vi "Handle Last Ack Core.vi"(4 "error in (no error)":errorcluster, 6 "Last Ack":refnum<class "Last Ack.lvclass">, 7 "Assert Startup UI in":refnum<class "Assert Startup UI.lvclass">) -> (0 "error out":errorcluster, 3 "Assert Startup UI out":refnum<class "Assert Startup UI.lvclass">)   [LabVIEW 2016, in "Assert Startup UI.lvlib" / "Assert Startup UI.lvclass"]
doc: "(<B>Filename</B>: Actor Framework.lvlib:Actor.lvclass:Handle Last Ack Core.vi)\n\nDefines how the caller actor responds to the Last Ack message from a nested actor. The Last Ack message is the final message a nested actor sends to its caller before it shuts down. The message contains information about the final state of the nested actor.\n\nBy default, this method does nothing except return any error the nested actor sent. A descendant class may override this method to define behavior."
uses:
  Assert Startup UI.lvclass
  <vilib>/ActorFramework/LastAck/Last Ack.lvclass
  Assert Startup UI.lvclass/Assert Startup UI.ctl
  Base UI Actor/Base UI Actor/Base UI Actor.lvclass
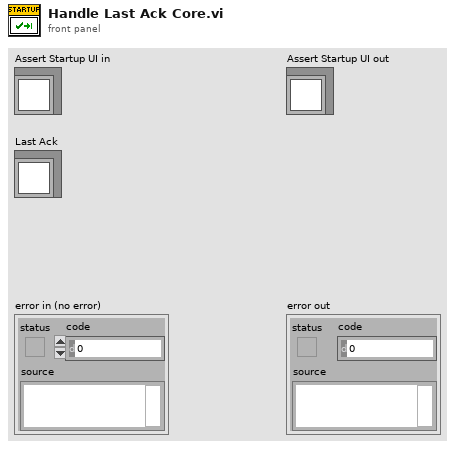
[diagram p1: front panel]
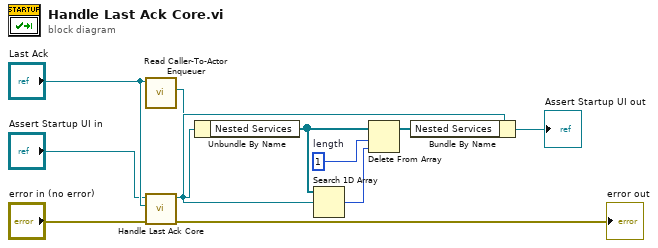
[diagram p0: block diagram]
diagram:
  w4 = 1  # length
  n1 = call <vilib>:"Read Caller-To-Actor Enqueuer.vi"("Last Ack"="Last Ack") -> ("Caller-to-Actor Enqueuer"=w6:refnum<class "Message Enqueuer.lvclass">)  [unwired: 10 in]
  n2 = call-parent "Handle Last Ack Core.vi"("error in (no error)"="error in (no error)", "Last Ack"="Last Ack", "Actor in"="Assert Startup UI in") -> ("error out"=→"error out":errorcluster, "Actor out"=w7:refnum<class "Assert Startup UI.lvclass">)  [unwired: 3 in]
  n3 = Unbundle By Name(w7) -> ("Nested Services"=w5:refnum<class "Message Enqueuer.lvclass">[])
  n4 = Search 1D Array(1D array=w5, element=w6) -> (index of element=w3:i32)  [unwired: 1 in]
  n5 = Delete From Array(array=w5, length=w4, index=w3) -> (array with subset deleted=w1:refnum<class "Message Enqueuer.lvclass">[])  [unwired: 1 out]
  n6 = Bundle By Name(cluster=w7, "Nested Services"=w1) -> (→"Assert Startup UI out":refnum<class "Assert Startup UI.lvclass">)
